vi "获取批次信息.vi"(8 "error in (no error)":errorcluster caption="错误输入（无错误）", 10 "产品型号":string, 11 "Tbl引用句柄":refnum<vi>) -> (0 "error out":errorcluster, 3 "引用输出":refnum<vi>)   [LabVIEW 2018]
uses:
  <vilib>/addons/database/Connection.llb/DB Tools Open Connec (String).vi
  <vilib>/addons/database/Connection.llb/Conn Execute.vi
  <vilib>/addons/database/Recordset.llb/Rec Fetch Recordset Data (R).vi
  <vilib>/addons/database/Recordset.llb/Rec Destroy - Connection.vi
  <vilib>/addons/database/NI_Database_API.lvlib
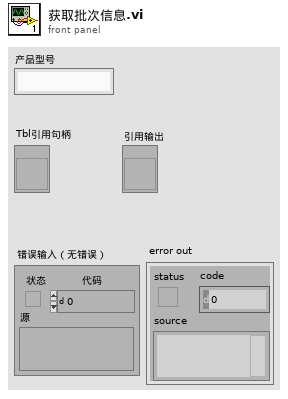
[diagram p1: front panel]
types:
  T1 = typedef "NI_Database_API.lvlib/Conn ObjectReference.ctl" = refnum<k1>
  T2 = typedef "NI_Database_API.lvlib/Rec ObjectReference.ctl" = refnum<k1>
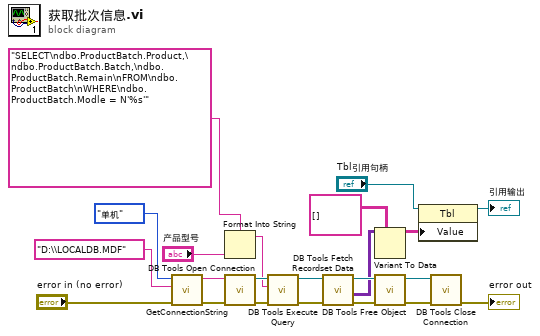
[diagram p0: block diagram]
diagram:
  n1 = call "GetConnectionString.vi"("error in (no error)"="error in (no error)", "Database Name"="D:\\LOCALDB.MDF", "连接模式"=enum16{"单机", "联网"}."单机") -> ("error out"=w20:errorcluster, "连接字符串"=w19:string)  [unwired: 3 in]
  n2 = Format Into String(format string="SELECT\ndbo.ProductBatch.Product,\ndbo.ProductBatch.Batch,\ndbo.ProductBatch.Remain\nFROM\ndbo.ProductBatch\nWHERE\ndbo.ProductBatch.Modle = N'%s'" ("SQL query"), "产品型号") -> (resulting string=w10:string)  [unwired: 2 in, 1 out]
  n3 = call-poly <vilib>:"DB Tools Open Connection.vi"("error in (no error)"=w20, "connection information"=w19) -> ("error out"=w18:errorcluster, "connection reference"=w17:T1)  [unwired: 6 in]
  n4 = call-poly <vilib>:"DB Tools Execute Query.vi"("error in (no error)"=w18, "SQL query"=w10, "connection reference"=w17) -> ("error out"=w16:errorcluster, "recordset reference"=w15:T2)  [unwired: 5 in]
  n5 = call-poly <vilib>:"DB Tools Fetch Recordset Data.vi"("error in (no error)"=w16, "recordset reference"=w15) -> ("error out"=w13:errorcluster, "recordset data"=w7:variant[][], "recordset reference out"=w14:T2)  [unwired: 3 in]
  n6 = Variant To Data(type=string[][] [] ("值"), Variant=w7) -> (data=w6:string[][])  [unwired: 1 in, 1 out]
  n7 = call-poly <vilib>:"DB Tools Free Object.vi"("error in (no error)"=w13, "recordset reference"=w14) -> ("error out"=w5:errorcluster, "connection reference"=w4:T1)  [unwired: 8 in]
  n8 = property class="Tbl"(reference="Tbl引用句柄", "Value"=w6) -> (reference out=→"引用输出":refnum<vi>)  [unwired: 1 in, 1 out]
  n9 = call <vilib>:"DB Tools Close Connection.vi"("error in (no error)"=w5, "connection reference"=w4) -> ("error out"=→"error out":errorcluster)  [unwired: 5 in]
